vi "LWXPS_PositionerCompensationPreFeedForwardSpatialNotchFilterGet.vi"(0 "XPS Reference IN":refnum<k24>, 5 "Positioner Name":string, 9 "Spatial Notch Number":i32, 11 "LabVIEW error IN":errorcluster) -> (3 "XPS Reference OUT":refnum<k24>, 4 "Returned error code":i32, 6 "Spatial Notch Step":dbl, 8 "Spatial Notch Bandwidth":dbl, 10 "Spatial Notch Gain":dbl, 14 "LabVIEW error OUT":errorcluster, 15 "XPS Error String":string)   [LabVIEW 2014]
uses:
  D:/XPSQ8_LabView_Library/Development/Source/Dll/Newport.XPS.CommandInterface.dll
  Dll/Newport.XPS.CommandInterface.dll
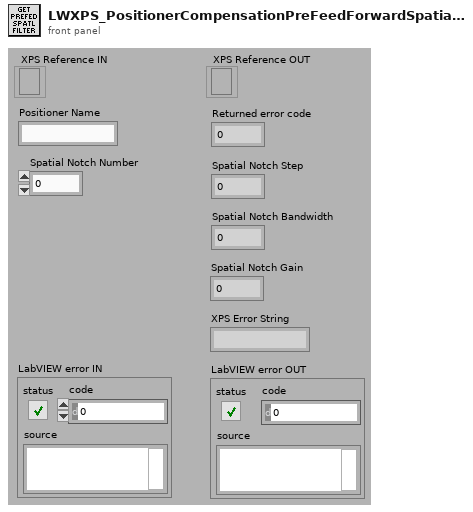
[diagram p1: front panel]
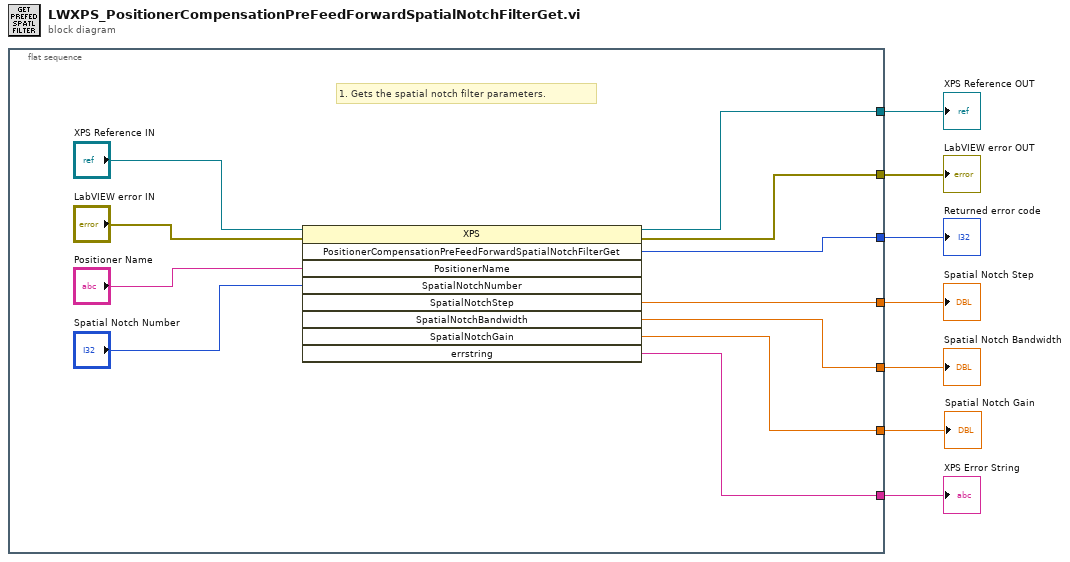
[diagram p0: block diagram]
diagram:
  n1 = flat-sequence {
    tunnel: [w16] -> w7
    tunnel: [w10] -> w6
    tunnel: [w17] -> w5
    tunnel: [w13] -> w4
    tunnel: [w12] -> w3
    tunnel: [w8] -> w2
    tunnel: [w11] -> w1
    frame #0 {
      # "1. Gets the spatial notch filter parameters."
      n2 = invoke class="XPS" method="PositionerCompensationPreFeedForwardSpatialNotchFilterGet"(reference="XPS Reference IN", error in="LabVIEW error IN", "PositionerName"="Positioner Name", "SpatialNotchNumber"="Spatial Notch Number") -> (reference out=w16:refnum<k24>, error out=w10:errorcluster, "PositionerCompensationPreFeedForwardSpatialNotchFilterGet"=w17:i32, "SpatialNotchStep"=w13:dbl, "SpatialNotchBandwidth"=w12:dbl, "SpatialNotchGain"=w11:dbl, "errstring"=w8:string)  [unwired: 5 in, 2 out]
    }
  }
  "XPS Error String" <- w2
  "XPS Reference OUT" <- w7
  "LabVIEW error OUT" <- w6
  "Returned error code" <- w5
  "Spatial Notch Step" <- w4
  "Spatial Notch Bandwidth" <- w3
  "Spatial Notch Gain" <- w1
